vi "CameraSetScaledAttrBrightness.vi"(8 "error in":errorcluster, 9 "Scaled":dbl, 10 "Attr String":string, 11 "IMAQdx Session in":T1) -> (0 "error out":errorcluster, 3 "IMAQdx Session":T1)   [LabVIEW 2025]
doc: "This VI updates an attribute where input unit is percentage and camera parameter may be in another unit.\n\nThis software is licensed. Open the labview\\readme\\WPI Robotics Library Open Source License.txt file for more information."
uses:
  <vilib>/userDefined/High Color/IMAQdx.ctl
  <resource>/objmgr/imaqdx.rc
  <vilib>/gmath/NI_Gmath.lvlib
panel:
  out "MaxDBL":dbl
  out "MinDBL":dbl
  out "element":dbl
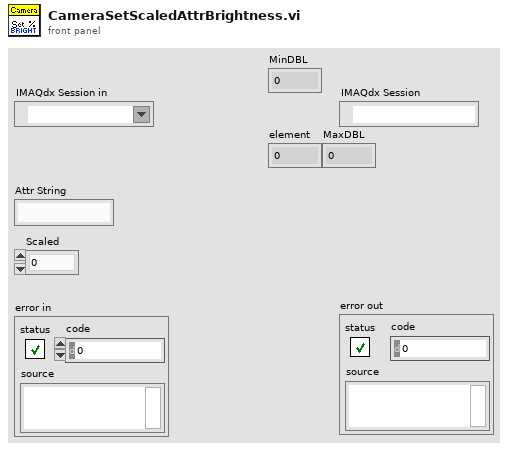
[diagram p1: front panel]
types:
  T1 = typedef "IMAQdx.ctl" = refnum<k21>
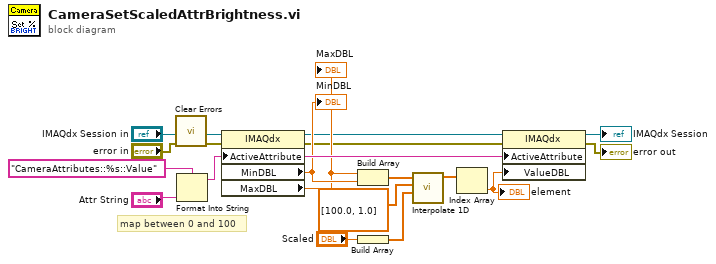
[diagram p0: block diagram]
diagram:
  # "map between 0 and 100"
  n1 = call <vilib>:"Clear Errors.vi"("error in (no error)"="error in") -> ("error out"=w1:errorcluster)  [unwired: 5 in, 1 out]
  n2 = Format Into String(format string="CameraAttributes::%s::Value" ("Attr Format"), "Attr String") -> (resulting string=w8:string)  [unwired: 2 in, 1 out]
  n3 = property class="IMAQdx"(reference="IMAQdx Session in", error in=w1, "ActiveAttribute"=w8) -> (reference out=w4:T1, error out=w2:errorcluster, "MinDBL"=w7:dbl, "MaxDBL"=w6:dbl)
  "MinDBL" <- w7
  "MaxDBL" <- w6
  n4 = Build Array(w6, w7) -> (w14:dbl[])
  n5 = Build Array("Scaled") -> (w11:dbl[])
  n6 = call <vilib>:"Interpolate 1D.vi"("xi"=w11, "X"=dbl[] [100.0, 1.0], "Y"=w14) -> ("yi"=w10:dbl[])  [unwired: 6 in, 2 out]
  n7 = Index Array(array=w10) -> (element=w9:dbl)  [unwired: 1 in]
  "element" <- w9
  n8 = property class="IMAQdx"(reference=w4, error in=w2, "ActiveAttribute"=w8, "ValueDBL"=w9) -> (reference out=→"IMAQdx Session":T1, error out=→"error out":errorcluster)
